vi "Write Nil by Reference.vi"(8 "Error In":errorcluster, 11 "Writer In":refnum<data-value>) -> (0 "Error Out":errorcluster, 3 "Writer Out":refnum<data-value>)   [LabVIEW 2018, in "Toolkit.lvlib" / "Writer.lvclass"]
uses:
  Writer.lvclass
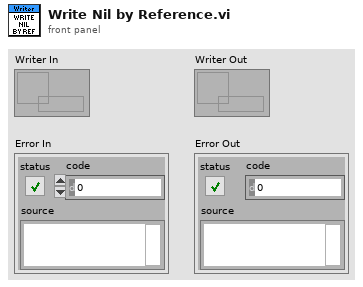
[diagram p1: front panel]
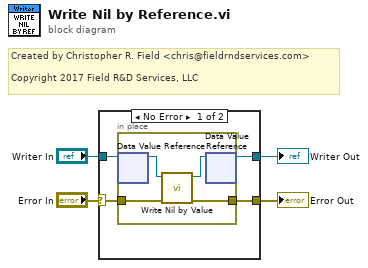
[diagram p0: block diagram]
diagram:
  # "Created by Christopher R. Field <chris@fieldrndservices.com>\n\nCopyright 2017 Field R&D Services, LLC"
  n1 = case shown="No Error" "Error In" {
    selector: "Error In" -> [w6 w14]
    tunnel: [w5 w14] -> w3
    tunnel: "Writer In" -> [w8 w13]
    tunnel: [w7 w13] -> w1
    frame No Error {
      n2 = in-place {
        in-place-border: w6 -> [w10]
        in-place-border: [w9] -> w5
        n3 = in-place-dvr #1(w8) -> (w12:refnum<class "Writer.lvclass">)  [unwired: 1 out]
        n4 = call "Write Nil by Value.vi"("Error In"=w10, "Writer In"=w12) -> ("Error Out"=w9:errorcluster, "Writer Out"=w11:refnum<class "Writer.lvclass">)  [unwired: 8 in]
        n5 = in-place-dvr #1(w11) -> (w7:refnum<data-value>)  [unwired: 1 out]
      }
    }
    frame Error {
    }
  }
  "Error Out" <- w3
  "Writer Out" <- w1
